vi "PrjPath_Save.vi"(7 "error in (no error)":errorcluster caption="错误输入（无错误）", 9 "Path":path) -> (0 "error out":errorcluster caption="错误输出")   [LabVIEW 2016]
uses:
  <vilib>/Utility/config.llb/Write Key (Path).vi
  <vilib>/Utility/config.llb/NI_LVConfig.lvlib
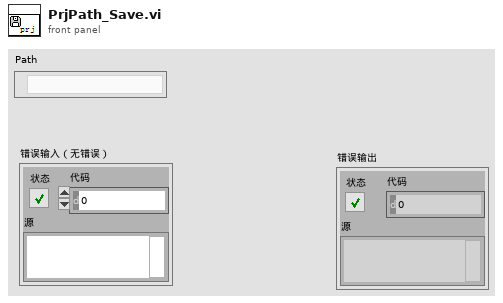
[diagram p1: front panel]
types:
  T1 = cluster{"TREE PNG":path, "User Guide":path, "DefaultSave":path, "BuildPath":path, "Image":path, "Modules":path, "Configuration":path, "License":path, "SplitFiles":path, "System.ini":path}
  T2 = typedef "NI_LVConfig.lvlib/Config Data RefNum.ctl" = refnum<k1>
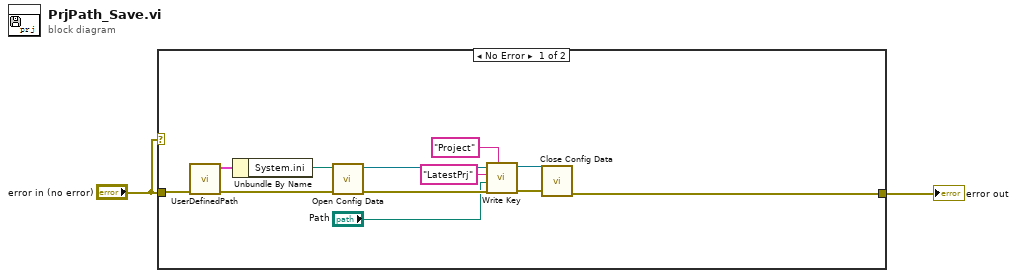
[diagram p0: block diagram]
diagram:
  n1 = case shown="No Error" "error in (no error)" {
    tunnel: [w4 w14] -> w2
    tunnel: "error in (no error)" -> [w5 w14]
    frame No Error {
      n2 = call "UserDefinedPath.vi"() -> ("UserDefinedPath"=w13:T1)  [unwired: 11 in]
      n3 = Unbundle By Name(w13) -> ("System.ini"=w12:path)
      n4 = call <vilib>:"Open Config Data.vi"("error in (no error)"=w5, "configuration file path"=w12) -> ("error out"=w10:errorcluster, "refnum"=w11:T2)  [unwired: 7 in, 1 out]
      n5 = call-poly <vilib>:"Write Key.vi"("section"="Project", "error in (no error)"=w10, "value"="Path", "key"="LatestPrj", "refnum"=w11) -> ("error out"=w8:errorcluster, "refnum out"=w9:T2)  [unwired: 4 in, 1 out]
      n6 = call <vilib>:"Close Config Data.vi"("error in (no error)"=w8, "refnum"=w9) -> ("error out"=w4:errorcluster)  [unwired: 8 in, 1 out]
    }
    frame Error {
    }
  }
  "error out" <- w2
